vi "startHW.vi"(8 "error in (no error)":errorcluster, 11 "Target in":refnum<class "Target.lvclass">) -> (0 "error out":errorcluster, 3 "Target out":refnum<class "Target.lvclass">)   [LabVIEW 2012, in "Target.lvclass"]
doc: "Performs any operations necessary to start the hardware."
uses:
  Target.lvclass
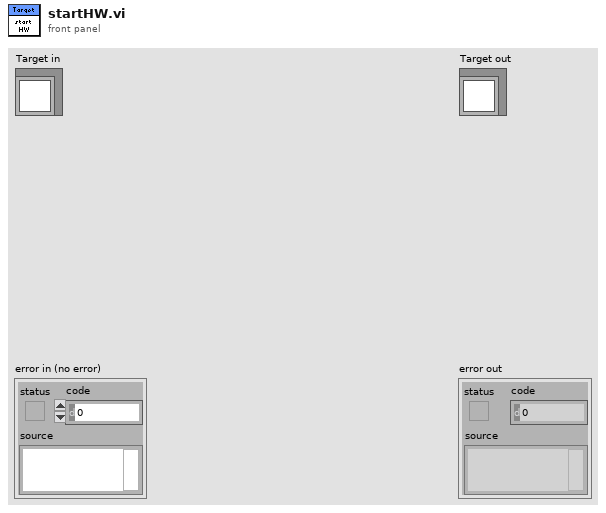
[diagram p1: front panel]
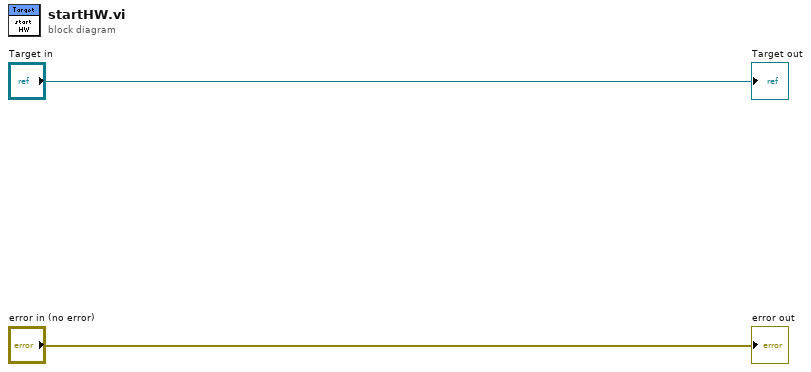
[diagram p0: block diagram]
diagram:
  "error out" <- "error in (no error)"
  "Target out" <- "Target in"
